vi "Keithley 6514 Trigger Layer Config.vi"(0 "Resource In":refnum<visa-resource-name>, 1 "Check For SCPI Errors? (T)":bool=TRUE, 2 "output trigger (sense:T)":bool=TRUE, 3 "async trigger link output (line 2:2)":u16(ring)=2 items=["line 1"=1, "line 2"=2, "line 3"=3, "line 4"=4, "line 5"=5, "line 6"=6], 5 "direction (acceptor:F)":bool, 7 "count (set:0)":u16(ring) items=["set  value", "infinite", "min", "max"], 9 "count value (1)":i16=1 min=1 max=2500 step=1, 11 "error in (no error)":T1, 12 "source (imm:0)":u16(ring) items=["immediate", "trigger link"], 13 "delay (secs) (0)":dbl min=0.0 max=999.9999 format="%.3f", 14 "async trigger link input (line 1:1)":u16(ring)=1 items=["line 1"=1, "line 2"=2, "line 3"=3, "line 4"=4, "line 5"=5, "line 6"=6]) -> (4 "Resource Out (dupl)":refnum<visa-resource-name>, 15 "error out":T1)   [LabVIEW 2014, in "KE6514Driver.lvlib"]
doc: "This VI is used to configure the settings for the Measure Layer (Trigger) of the trigger model. \n\ncount:\n0 = Set Value\n1 = Inifinite\n2 = min\n3 = max\n\nsource:\n0 = Immediate\n1 = Tlink\n\ndirection:\nFALSE= acceptor\nTRUE = source\n\nCount Value:\n1 to 2500\n\nDelay:\n0.001 to 999.9999 seconds\n\nOutput Trigger:\nFALSE = none\nTRUE = Sense\n\nAsync Trigger Link Input:\n1 = Line 1\n2 = Line 2\n3 = Line 3\n4 = Line 4\n5 = Line 5\n6 = Line 6\n\nAsync Trigger Link Output:\n1 = Line 1\n2 = Line 2\n3 = Line 3\n4 = Line 4\n5 = Line 5\n6 = Line 6"
uses:
  KE6514Driver.lvlib
panel:
  # "source\nacceptor"
  # "sense\nnone"
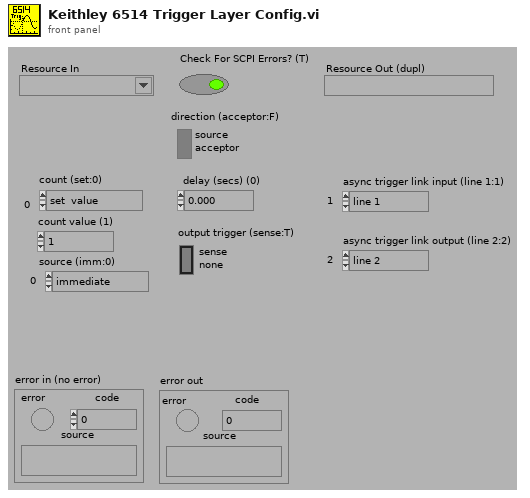
[diagram p1: front panel]
types:
  T1 = cluster{"error":bool, "code":i32, "source":string}
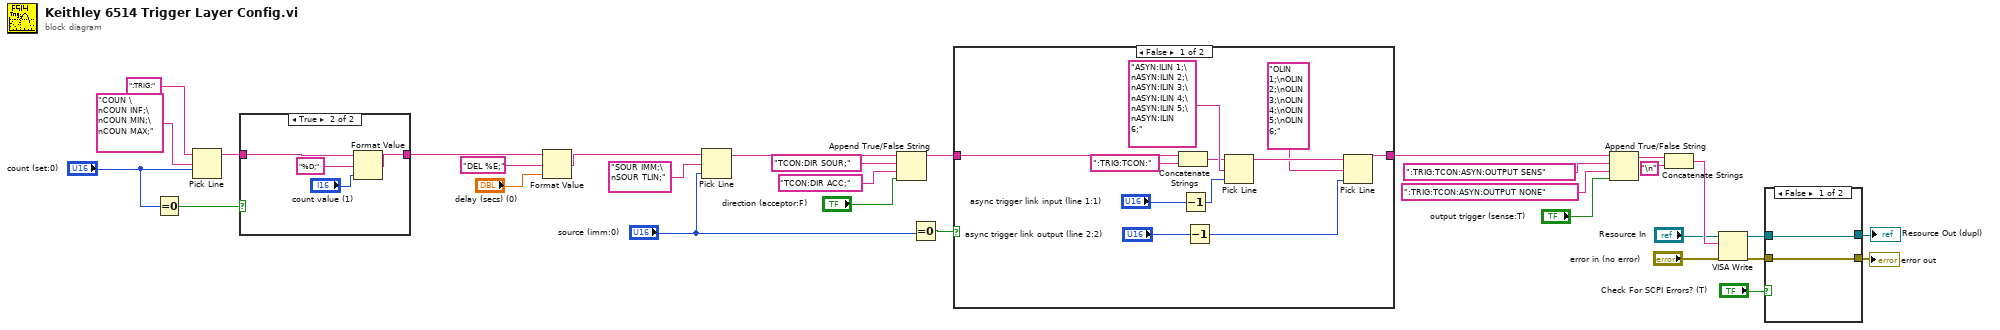
[diagram p0: block diagram]
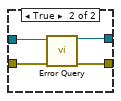
[diagram p2: hidden frame]
diagram:
  n1 = Equal To 0?(x="count (set:0)") -> (x = 0?=w29:bool)
  n2 = Pick Line(string ("")=":TRIG:", multi-line string="COUN \nCOUN INF;\nCOUN MIN;\nCOUN MAX;", line index="count (set:0)") -> (output string=w17:string)
  n3 = case shown="True" w29 {
    tunnel: w17 -> [w32 w35]
    tunnel: [w32 w33] -> w16
    frame False {
    }
    frame True {
      n4 = Format Value(string ("")=w35, format string="%D;", value (0)="count value (1)") -> (output string=w33:string)
    }
  }
  n5 = Format Value(string ("")=w16, format string="DEL %E;", value (0)="delay (secs) (0)") -> (output string=w15:string)
  n6 = Pick Line(string ("")=w15, multi-line string="SOUR IMM;\nSOUR TLIN;", line index="source (imm:0)") -> (output string=w14:string)
  n7 = Append True/False String(1:"direction (acceptor:F)", 2:"TCON:DIR ACC;", 3:"TCON:DIR SOUR;", 4:w14) -> (0:w12:string)
  n8 = Equal To 0?(x="source (imm:0)") -> (x = 0?=w13:bool)
  n9 = case shown="False" w13 {
    tunnel: w12 -> [w42 w48]
    tunnel: [w37 w48] -> w11
    frame False {
      n10 = Concatenate Strings(w42, ":TRIG:TCON:") -> (w44:string)
      n11 = Decrement(x="async trigger link input (line 1:1)") -> (x-1=w40:u16)
      n12 = Decrement(x="async trigger link output (line 2:2)") -> (x-1=w38:u16)
      n13 = Pick Line(string ("")=w44, multi-line string="ASYN:ILIN 1;\nASYN:ILIN 2;\nASYN:ILIN 3;\nASYN:ILIN 4;\nASYN:ILIN 5;\nASYN:ILIN 6;", line index=w40) -> (output string=w47:string)
      n14 = Pick Line(string ("")=w47, multi-line string="OLIN 1;\nOLIN 2;\nOLIN 3;\nOLIN 4;\nOLIN 5;\nOLIN 6;", line index=w38) -> (output string=w37:string)
    }
    frame True {
    }
  }
  n15 = Append True/False String(1:"output trigger (sense:T)", 2:":TRIG:TCON:ASYN:OUTPUT NONE", 3:":TRIG:TCON:ASYN:OUTPUT SENS", 4:w11) -> (0:w10:string)
  n16 = Concatenate Strings(w10, "\n") -> (w8:string)
  n17 = VISA Write(VISA resource name="Resource In", write buffer=w8, error in (no error)="error in (no error)") -> (VISA resource name out=w4:refnum<visa-resource-name>, error out=w3:errorcluster)  [unwired: 1 out]
  n18 = case shown="False" "Check For SCPI Errors? (T)" {
    tunnel: w4 -> [w50 w53]
    tunnel: w3 -> [w49 w54]
    tunnel: [w49 w52] -> w1
    tunnel: [w50 w51] -> w2
    frame False {
    }
    frame True {
      n19 = call "Error Query.vi"("VISA Resource In"=w53, "error in (no error)"=w54) -> ("VISA Resource Out (dupl)"=w51:refnum<visa-resource-name>, "error out"=w52:errorcluster)  [unwired: 10 in, 2 out]
    }
  }
  "error out" <- w1
  "Resource Out (dupl)" <- w2
